vi "begin direct read at least.vi"(7 "id":u32, 8 "error in":errorcluster, 9 "max bytes to read":u32, 10 "min bytes to read":u32, 11 "connection in":refnum<class "connection.lvclass">) -> (0 "error out":errorcluster)   [LabVIEW 2016, in "connection.lvclass"]
uses:
  connection.lvclass
  connection.lvclass/connection.ctl
  dllwrapper/library path.vi
  <vilib>/Utility/error.llb/Error Cluster From Error Code.vi
  dllwrapper/async tls dl.lvlib
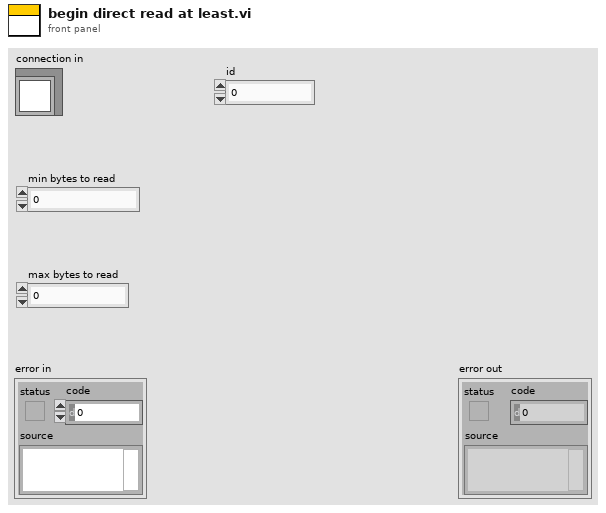
[diagram p1: front panel]
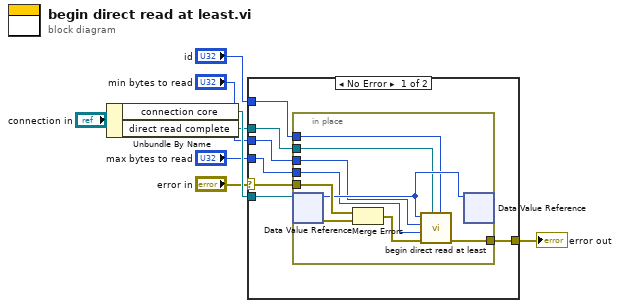
[diagram p0: block diagram]
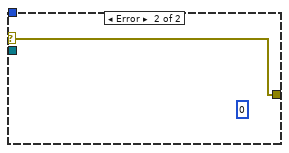
[diagram p2: hidden frame]
diagram:
  n1 = Unbundle By Name("connection in") -> ("connection core"=w7:refnum<data-value>, "direct read complete"=w4:refnum<user-event>)
  n2 = case shown="No Error" "error in" {
    selector: "error in" -> [w14 w25]
    tunnel: w7 -> [w15 _]
    tunnel: [w13 w25] -> w5
    tunnel: w4 -> [w12 _]
    tunnel: "id" -> [w11 _]
    tunnel: "max bytes to read" -> [w10 _]
    tunnel: "min bytes to read" -> [w9 _]
    frame No Error {
      n3 = in-place {
        in-place-border: w14 -> [w24]
        in-place-border: [w21] -> w13
        in-place-border: w12 -> [w19]
        in-place-border: w11 -> [w18]
        in-place-border: w10 -> [w17]
        in-place-border: w9 -> [w16]
        n4 = in-place-dvr #1(w15) -> (w20:u64, w23:errorcluster)
        n5 = Merge Errors(w24, w23) -> (w22:errorcluster)
        n6 = call "begin direct read at least.vi"("id"=w18, "event"=w19, "error in"=w22, "max bytes to read"=w17, "min bytes to read"=w16, "socket"=w20) -> ("error out"=w21:errorcluster)  [unwired: 5 in]
        n7 = in-place-dvr #1(w20) -> ()  [unwired: 2 out]
      }
    }
    frame Error {
      (unwired) u64 0 ("size")
    }
  }
  "error out" <- w5
